vi "Save.vi"(8 "error in (no error)":errorcluster, 9 "refnum in":refnum<file>, 10 "time stamp":timestamp, 11 "array":dbl[][](array[numeric])) -> (0 "error out":errorcluster, 1 "refnum out":refnum<file>)   [LabVIEW 2019]
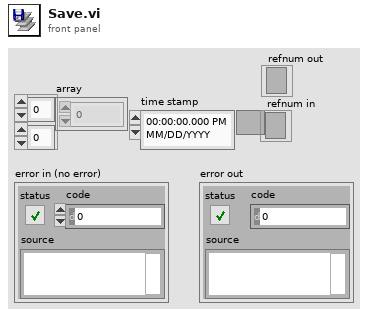
[diagram p1: front panel]
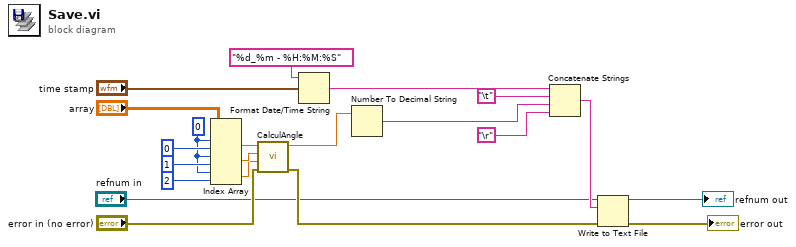
[diagram p0: block diagram]
diagram:
  w6 = 0 ("disabled index (row)")
  n1 = Index Array(array="array", index (row) #1=w6, index (col) #1=0 ("disabled index (col)"), index (row) #2=w6, index (col) #2=1 ("disabled index (col)"), index (row) #3=w6, index (col) #3=2 ("disabled index (col)")) -> (element #1=w21:dbl, element #2=w20:dbl, element #3=w19:dbl)
  n2 = call "CalculAngle.vi"("error constant"="error in (no error)", "Zaxis"=w19, "Yaxis"=w20, "Xaxis"=w21) -> ("error constant 2"=w5:errorcluster, "Numeric"=w13:dbl)  [unwired: 6 in]
  n3 = Format Date/Time String(time format string (%c)="%d_%m - %H:%M:%S", seconds (now)="time stamp") -> (date/time string=w16:string)  [unwired: 1 in]
  n4 = Number To Decimal String(number=w13) -> (decimal integer string=w14:string)  [unwired: 1 in]
  n5 = Concatenate Strings(w16, "\t", w14, "\r") -> (w10:string)
  n6 = Write to Text File(file (use dialog)="refnum in", text=w10, error in=w5) -> (refnum out=→"refnum out":refnum<file>, error out=→"error out":errorcluster)  [unwired: 1 in, 1 out]
